vi "FRCts20_Backend_API_Competition.vi"(8 "error in (no error)":errorcluster, 10 "Command":T1="GetCompetition", 11 "Competition In":T2) -> (0 "error out":errorcluster, 2 "Status":string, 3 "Competition Out":T2)   [LabVIEW 2014]
doc: "This VI is in charge of returning data about a selected competition, including all contained divisions."
uses:
  FRCts20_Backend_API_Competition.ctl
  FRCts20_Backend_API_Command_Competition.ctl
  FRCts20_Backend_FGVOperation.ctl
  FRCts20_Backend_Engine.lvlib
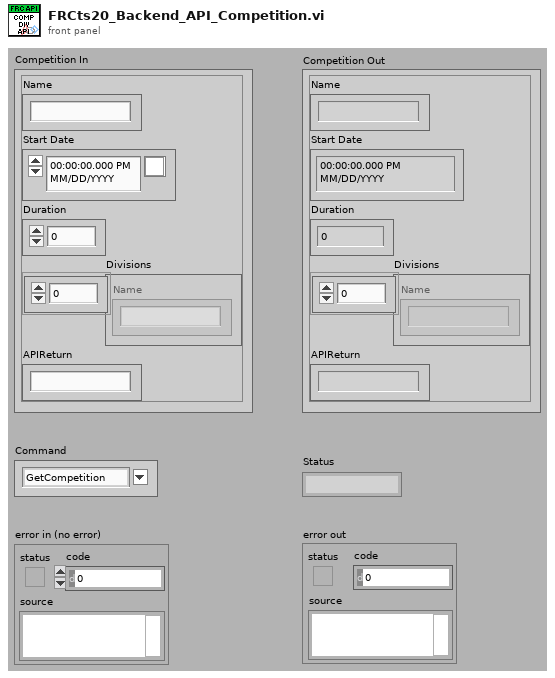
[diagram p1: front panel]
types:
  T1 = typedef "FRCts20_Backend_API_Command_Competition.ctl" = string
  T2 = typedef "FRCts20_Backend_API_Competition.ctl" = cluster{"Name":string, "Start Date":timestamp, "Duration":u8, "Divisions":string[], "APIReturn":string}
  T3 = typedef "FRCts20_Backend_Engine.lvlib/FRCts20_Backend_FGVOperation.ctl" = enum16{"Initialize", "EnqueueMessage", "EnqueueDataReturn", "FlushMessage", "FlushDataReturn"}
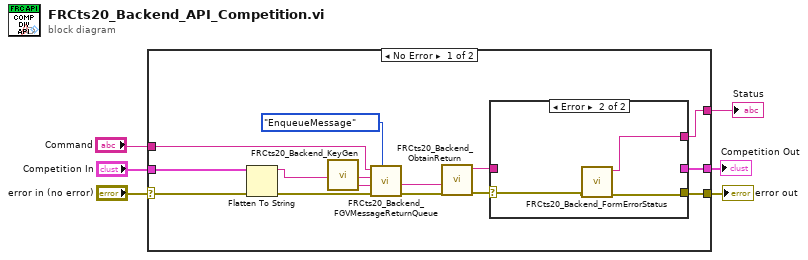
[diagram p0: block diagram]
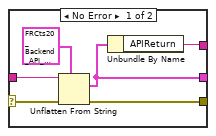
[diagram p2: hidden frame]
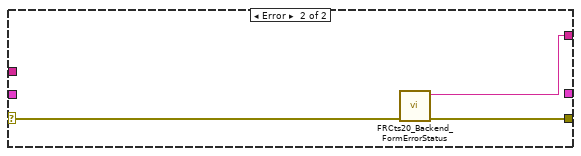
[diagram p3: hidden frame]
diagram:
  n1 = case shown="No Error" "error in (no error)" {
    selector: "error in (no error)" -> [w20 w32]
    tunnel: [w10 w31] -> w5
    tunnel: [w8 w30] -> w4
    tunnel: [w9 _] -> w3
    tunnel: "Competition In" -> [w13 _]
    tunnel: "Command" -> [w15 _]
    frame No Error {
      n2 = Flatten To String(anything=w13, error in (no error)=w20) -> (data string=w12:string, error out=w14:errorcluster)  [unwired: 2 in, 1 out]
      n3 = call "FRCts20_Backend_KeyGen.vi"() -> ("Keygen"=w19:string)  [unwired: 27 in]
      n4 = call "FRCts20_Backend_FGVMessageReturnQueue.vi"("Operation"=FRCts20_Backend_FGVOperation."EnqueueMessage", "error in (no error)"=w14, "Key"=w19, "Message Value"=w12, "Message Name"=w15) -> ("error out"=w17:errorcluster, "Key (Duplicate)"=w16:string)  [unwired: 5 in]
      n5 = call "FRCts20_Backend_ObtainReturn.vi"("error in (no error)"=w17, "Key"=w16) -> ("error out"=w11:errorcluster, "Message Value"=w7:string)  [unwired: 8 in]
      n6 = case shown="Error" w11 {
        selector: w11 -> [w25 w28]
        tunnel: [w26 w29] -> w10
        tunnel: [w24 _] -> w9
        tunnel: [w23 w27] -> w8
        tunnel: w7 -> [w21 _]
        frame No Error {
          n7 = Unflatten From String(type=T2 {"Name"="", "Start Date"=timestamp(0 s since 1904-01-01), "Duration"=0, "Divisions"=[], "APIReturn"=""} ("Competition"), binary string=w21, error in (no error)=w25) -> (value=w24:T2, error out=w26:errorcluster)  [unwired: 2 in, 1 out]
          n8 = Unbundle By Name(w24) -> ("APIReturn"=w23:string)
        }
        frame Error {
          n9 = call "FRCts20_Backend_FormErrorStatus.vi"("error in (no error)"=w28) -> ("error out"=w29:errorcluster, "String"=w27:string)  [unwired: 9 in]
        }
      }
    }
    frame Error {
      n10 = call "FRCts20_Backend_FormErrorStatus.vi"("error in (no error)"=w32) -> ("error out"=w31:errorcluster, "String"=w30:string)  [unwired: 9 in]
    }
  }
  "error out" <- w5
  "Status" <- w4
  "Competition Out" <- w3
